vi "Write Plugin Options.vi"(8 "error in (no error)":errorcluster, 10 "Plugin Options":T1, 11 "MeasurementMetaData in":refnum<class "MeasurementMetaData.lvclass">) -> (0 "error out":errorcluster, 3 "MeasurementMetaData out":refnum<class "MeasurementMetaData.lvclass">)   [LabVIEW 2013, in "MeasurementMetaData.lvclass"]
uses:
  MeasurementMetaData.lvclass
  Plugin Settings.ctl
  MeasurementMetaData.lvclass/MeasurementMetaData.ctl
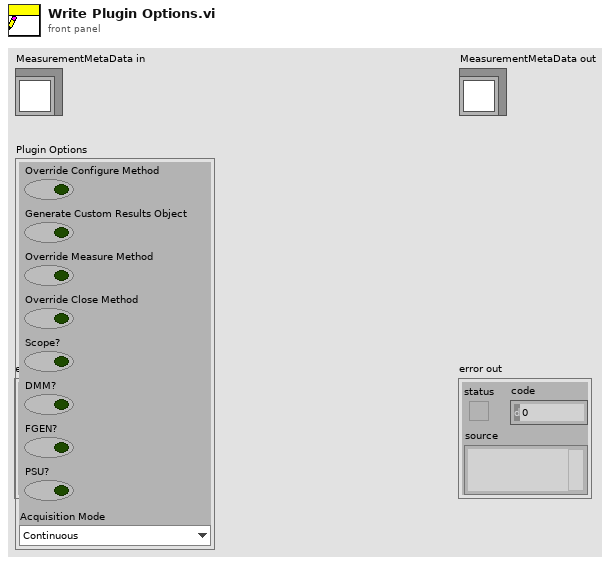
[diagram p1: front panel]
types:
  T1 = typedef "MeasurementMetaData.lvclass/Plugin Settings.ctl" = cluster{"Override Configure Method":bool, "Generate Custom Results Object":bool, "Override Measure Method":bool, "Override Close Method":bool, "Scope?":bool, "DMM?":bool, "FGEN?":bool, "PSU?":bool, "Acquisition Mode":enum16{"Continuous", "Single-Shot"}}
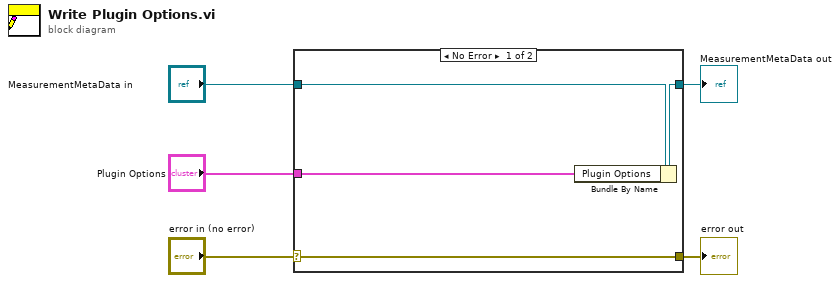
[diagram p0: block diagram]
diagram:
  n1 = case shown="No Error" "error in (no error)" {
    selector: "error in (no error)" -> [w9 w10]
    tunnel: [w9 w10] -> w4
    tunnel: [w7 w11] -> w2
    tunnel: "MeasurementMetaData in" -> [w8 w11]
    tunnel: "Plugin Options" -> [w6 _]
    frame No Error {
      n2 = Bundle By Name(cluster=w8, "Plugin Options"=w6) -> (w7:refnum<class "MeasurementMetaData.lvclass">)
    }
    frame Error {
    }
  }
  "error out" <- w4
  "MeasurementMetaData out" <- w2
